vi "Configure Digital Channel.vi"(5 "Enable Digital Channel (T: Enable)":bool=TRUE, 6 "Threshold (1.4 v)":dbl=1.4, 7 "Digital Channel (0: Digital Channel 0)":u8(ring) items=["Digital Channel 0", "Digital Channel 1", "Digital Channel 2", "Digital Channel 3", "Digital Channel 4", "Digital Channel 5", "Digital Channel 6", "Digital Channel 7", "Digital Channel 8", "Digital Channel 9", "Digital Channel 10", "Digital Channel 11", "Digital Channel 12", "Digital Channel 13", "Digital Channel 14", "Digital Channel 15"], 8 "error in (no error)":errorcluster, 9 "CQ Threshold (1.4 v)":dbl=1.4, 10 "CQ Channel (0: CQ Channel 0)":u8(ring) items=["CQ Channel 0"], 11 "VISA resource name":refnum<visa-resource-name>) -> (0 "error out":errorcluster, 3 "VISA resource name out":refnum<visa-resource-name>)   [LabVIEW 2015, in "Tektronix 7000 Series.lvlib"]
doc: "Configures the threshold of an oscilloscope for a specified channel. This VI also configures threshold for CQ0.\n\n<B>Note:</B> \nThese commands are not supported by TDS or CSA models."
uses:
  <instrlib>/Tektronix 7000 Series/Tektronix 7000 Series.lvlib
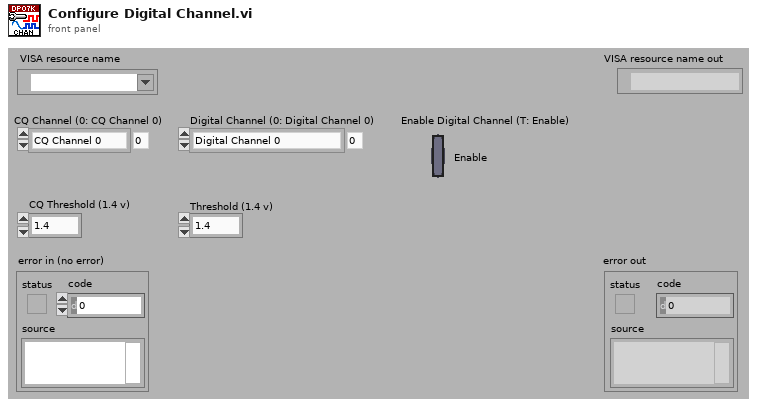
[diagram p1: front panel]
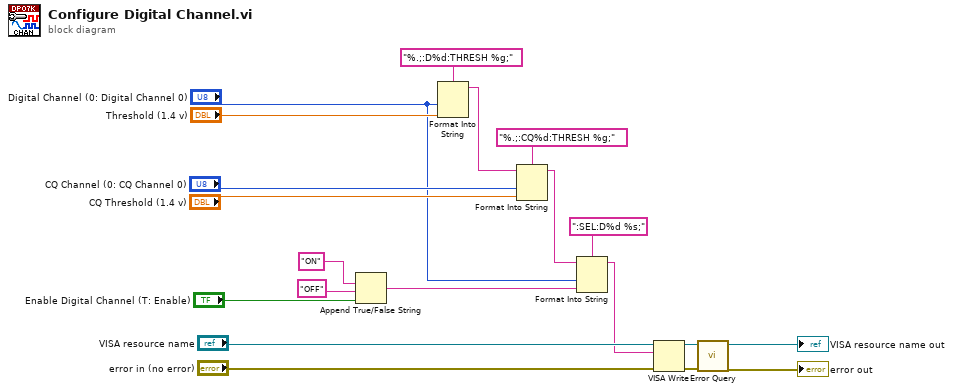
[diagram p0: block diagram]
diagram:
  n1 = Append True/False String(1:"Enable Digital Channel (T: Enable)", 2:"OFF", 3:"ON") -> (0:w1:string)  [unwired: 1 out]
  n2 = Format Into String(format string="%.;:D%d:THRESH %g;", "Digital Channel (0: Digital Channel 0)", "Threshold (1.4 v)") -> (resulting string=w18:string)  [unwired: 2 in, 1 out]
  n3 = Format Into String(format string="%.;:CQ%d:THRESH %g;", initial string=w18, "CQ Channel (0: CQ Channel 0)", "CQ Threshold (1.4 v)") -> (resulting string=w8:string)  [unwired: 1 in, 1 out]
  n4 = Format Into String(format string=":SEL:D%d %s;", initial string=w8, "Digital Channel (0: Digital Channel 0)", w1) -> (resulting string=w5:string)  [unwired: 1 in, 1 out]
  n5 = VISA Write(VISA resource name="VISA resource name", write buffer=w5, error in (no error)="error in (no error)") -> (VISA resource name out=w12:refnum<visa-resource-name>, error out=w11:errorcluster)  [unwired: 1 out]
  n6 = call <instrlib>:"Error Query.vi"("error in (no error)"=w11, "VISA resource name"=w12) -> ("error out"=→"error out":errorcluster, "VISA resource name out"=→"VISA resource name out":refnum<visa-resource-name>)  [unwired: 8 out]
